vi "PH_PSDBWriter.read out PHELIX Subsystems.vi"(4 "Config DB Subsystem":string="N/A") -> (0 "Metadata.Data Status":T1 items=["no info", "no Data collection", "no problem", "Error getting the ID", "Error writing Data", "Error getting the subsystem", "Error getting the Shot ID", "Error getting the Shot Types", "Error getting the Experiments", "Error verifying wanted Shottype", "Error verifying wanted Experiment"], 1 "Metadata.Subsystem":T2 caption="PHELIX Subsysteme" items=["Miscellaneous", "fs-Frontend", "ns-Frontend", "PreAmp", "MainAmp", "MAS", "COS", "Beamline", "Experiment Laserbay", "Experiment Laserlabor", "Experiment Z6", "Timing", "Pulsed Power"], 2 "Subsystem":string)   [LabVIEW 2014, in "PH_PSDBWriter.lvlib"]
doc: "This VI gets the subystem out of the string entry from the configuration database."
uses:
  PH_PSDBWriter.lvlib
  PH_PSDBWriter.PHELIX-Subsystems.ctl
  PH_PSDBWriter.Data Status.ctl
panel:
  in  "PHELIX Subsystems":T2 caption="PHELIX Subsysteme" items=["Miscellaneous", "fs-Frontend", "ns-Frontend", "PreAmp", "MainAmp", "MAS", "COS", "Beamline", "Experiment Laserbay", "Experiment Laserlabor", "Experiment Z6", "Timing", "Pulsed Power"]
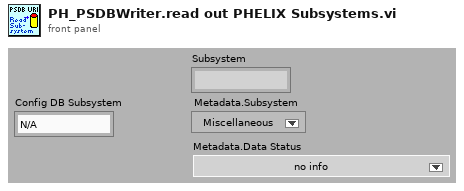
[diagram p1: front panel]
types:
  T1 = typedef "PH_PSDBWriter.lvlib/PH_PSDBWriter.Data Status.ctl" = i16
  T2 = typedef "PH_PSDBWriter.lvlib/PH_PSDBWriter.PHELIX-Subsystems.ctl" = i32
  T3 = typedef "LVStringsAndValuesArrayTypeDef_I32.ctl" = cluster{"String":string, "Value":i32}[]
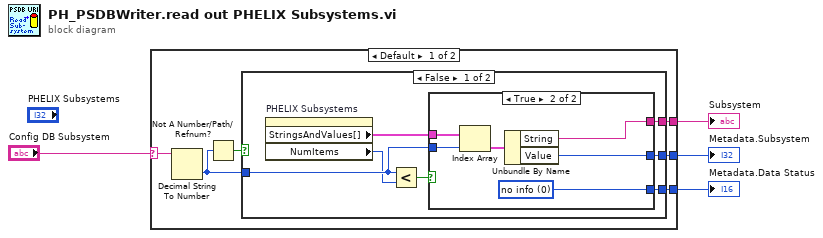
[diagram p0: block diagram]
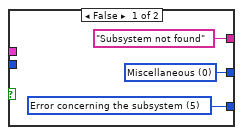
[diagram p2: hidden frame]
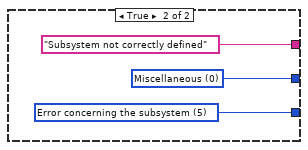
[diagram p3: hidden frame]
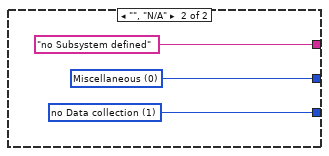
[diagram p4: hidden frame]
diagram:
  n1 = case shown="Default" "Config DB Subsystem" {
    selector: "Config DB Subsystem" -> [w10 _]
    tunnel: [w8 w32] -> w2
    tunnel: [w9 w31] -> w4
    tunnel: [w7 "no Subsystem defined" ("String")] -> w1
    frame Default {
      n2 = Decimal String To Number(string=w10) -> (number=w6:i32)  [unwired: 2 in, 1 out]
      n3 = Not A Number/Path/Refnum?(number/path/refnum=w6) -> (NaN/Path/Refnum?=w5:bool)
      n4 = case shown="False" w5 {
        tunnel: [w14 w27] -> w9
        tunnel: [w13 w28] -> w8
        tunnel: [w15 "Subsystem not correctly defined" ("t")] -> w7
        tunnel: w6 -> [w17 _]
        frame False {
          n5 = property on="PHELIX Subsystems" class="Ring (strict)"() -> ("StringsAndValues[]"=w12:T3, "NumItems"=w11:u32)  [unwired: 2 in, 2 out]
          n6 = Less?(x=w17, y=w11) -> (x < y?=w16:bool)
          n7 = case shown="True" w16 {
            tunnel: w12 -> [_ w26]
            tunnel: w17 -> [_ w24]
            tunnel: ["Subsystem not found" ("t") w23] -> w15
            tunnel: [w18 w22] -> w14
            tunnel: [w20 w21] -> w13
            frame False {
              w18 = T2 0 items=["Miscellaneous", "fs-Frontend", "ns-Frontend", "PreAmp", "MainAmp", "MAS", "COS", "Beamline", "Experiment Laserbay", "Experiment Laserlabor", "Experiment Z6"] ("Metadata.Subsystem")
              w20 = T1 5 items=["no info", "no Data collection", "no problem", "Error getting the instance ID", "Error writing Data to data base", "Error concerning the subsystem"] ("Metadata.Data Status")
            }
            frame True {
              w21 = T1 0 items=["no info", "no Data collection", "no problem", "Error getting the instance ID", "Error writing Data to data base"] ("Metadata.Data Status")
              n8 = Index Array(array=w26, index=w24) -> (element=w25:cluster{"String":string, "Value":i32})
              n9 = Unbundle By Name(w25) -> ("String"=w23:string, "Value"=w22:i32)
            }
          }
        }
        frame True {
          w27 = T2 0 items=["Miscellaneous", "fs-Frontend", "ns-Frontend", "PreAmp", "MainAmp", "MAS", "COS", "Beamline", "Experiment Laserbay", "Experiment Laserlabor", "Experiment Z6"] ("Metadata.Subsystem")
          w28 = T1 5 items=["no info", "no Data collection", "no problem", "Error getting the instance ID", "Error writing Data to data base", "Error concerning the subsystem"] ("Metadata.Data Status")
        }
      }
    }
    frame "", "N/A" {
      w31 = T2 0 items=["Miscellaneous", "fs-Frontend", "ns-Frontend", "PreAmp", "MainAmp", "MAS", "COS", "Beamline", "Experiment Laserbay", "Experiment Laserlabor", "Experiment Z6"] ("Metadata.Subsystem")
      w32 = T1 1 items=["no info", "no Data collection", "no problem", "Error getting the instance ID", "Error writing Data to data base"] ("Metadata.Data Status")
    }
  }
  "Metadata.Subsystem" <- w4
  "Metadata.Data Status" <- w2
  "Subsystem" <- w1
